vi "Build_Asylum_SetPISLoop.vi"(6 "outChannelString":string, 7 "whichLoop":i32, 8 "error in (no error)":errorcluster, 9 "PIS Controls":T1, 10 "inChannelString":string, 11 "eventString":string) -> (0 "error out":errorcluster, 3 "Command":string)   [LabVIEW 2019]
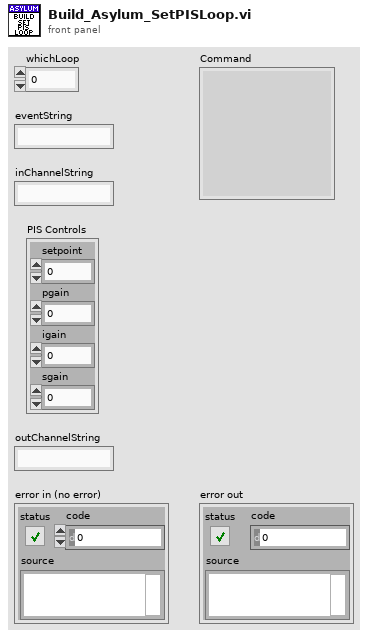
[diagram p1: front panel]
types:
  T1 = cluster{"setpoint":dbl, "pgain":dbl, "igain":dbl, "sgain":dbl}
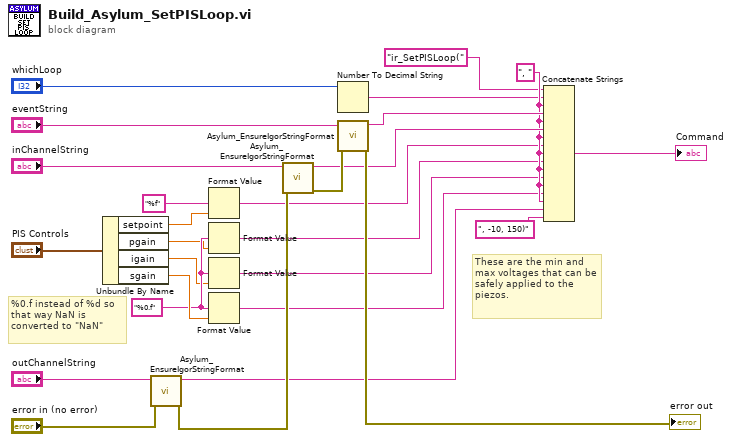
[diagram p0: block diagram]
diagram:
  w9 = "%0.f" ("format string")
  w18 = ", " ("string")
  # "%0.f instead of %d so that way NaN is converted to \"NaN\""
  # "These are the min and max voltages that can be safely applied to the piezos."
  n1 = Unbundle By Name("PIS Controls") -> ("setpoint"=w2:dbl, "pgain"=w7:dbl, "igain"=w8:dbl, "sgain"=w10:dbl)
  n2 = call "Asylum_EnsureIgorStringFormat.vi"("error in (no error)"="error in (no error)", "Value"="outChannelString") -> ("error out"=w27:errorcluster, "Value"=w23:string)  [unwired: 8 in]
  n3 = Format Value(format string="%f" ("Expected output Format"), value (0)=w2) -> (output string=w6:string)  [unwired: 1 in]
  n4 = Format Value(format string=w9, value (0)=w7) -> (output string=w5:string)  [unwired: 1 in]
  n5 = Format Value(format string=w9, value (0)=w8) -> (output string=w4:string)  [unwired: 1 in]
  n6 = Format Value(format string=w9, value (0)=w10) -> (output string=w3:string)  [unwired: 1 in]
  n7 = call "Asylum_EnsureIgorStringFormat.vi"("error in (no error)"=w27, "Value"="inChannelString") -> ("error out"=w25:errorcluster, "Value"=w22:string)  [unwired: 8 in]
  n8 = Number To Decimal String(number="whichLoop") -> (decimal integer string=w14:string)  [unwired: 1 in]
  n9 = call "Asylum_EnsureIgorStringFormat.vi"("error in (no error)"=w25, "Value"="eventString") -> ("error out"=→"error out":errorcluster, "Value"=w21:string)  [unwired: 8 in]
  n10 = Concatenate Strings("ir_SetPISLoop(" ("string"), w14, w18, w21, w18, w22, w18, w6, w18, w5, w18, w4, w18, w3, w18, w23, ", -10, 150)" ("string")) -> (→"Command":string)
